vi "VI Scripting with Structures - While Loop.vi"   [LabVIEW 2019]
doc: "This example contains sample code demonstrating common VI Scripting navigational tasks relating to While Loops."
panel:
  # "Overview: Illustrates several WhileLoop properties and methods used for inspecting and modifying While Loops with VI Scripting.\nInstructions:\nOpen the block diagram of this VI to see several examples of properties and methods related to While Loops and VI Scripting.\n\nNote: Browse the diagram of this example to learn about VI Scripting concepts. This example is not meant to be run."
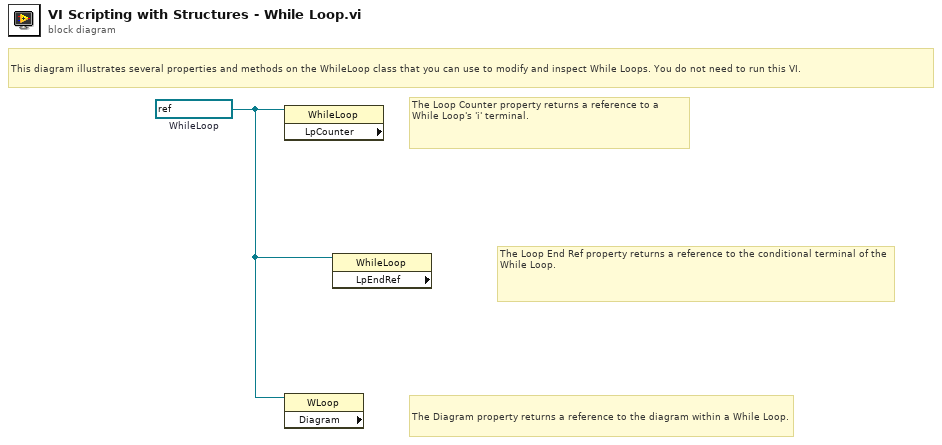
[diagram p0: block diagram]
diagram:
  w1 = refnum<vi> refnum  # WhileLoop
  # "The Diagram property returns a reference to the diagram within a While Loop."
  # "The Loop End Ref property returns a reference to the conditional terminal of the While Loop."
  # "The Loop Counter property returns a reference to a While Loop's 'i' terminal."
  # "This diagram illustrates several properties and methods on the WhileLoop class that you can use to modify and inspect While Loops. You do not need to run this VI."
  n1 = property class="WhileLoop" props=["LpCounter"](reference=w1) -> ()  [unwired: 1 in, 3 out]
  n2 = property class="WLoop" props=["Diagram"](reference=w1) -> ()  [unwired: 1 in, 3 out]
  n3 = property class="WhileLoop" props=["LpEndRef"](reference=w1) -> ()  [unwired: 1 in, 3 out]
